vi "Window-Stop funct acq dialogue.vi"(7 "Colour":u32(colorbox)=16777225, 8 "error in (no error)":errorcluster, 9 "Caption-Left button (Cancel)":string, 10 "Caption-Right button (OK)":string, 11 "Message string":string) -> (0 "error out":errorcluster, 1 "User canceled the Abort Or the func acqcompleted":bool, 3 "Funct acq completed":bool)   [LabVIEW 2013]
uses:
  <vilib>/Utility/miscctls.llb/LVPointTypeDef.ctl
  Typedefs/Set Main VI cursor.ctl
  Global Variables/General Globals.vi
panel:
  in  "Left Button":bool
  in  "Rigth Button":bool
  out "Message":string
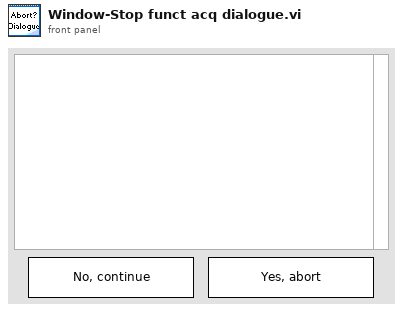
[diagram p1: front panel]
types:
  T1 = typedef "Set Main VI cursor.ctl" = enum16{"Release busy cursor", "Set busy cursor"}
  T2 = typedef "LVPointTypeDef.ctl" = cluster{"Horizontal":i16, "Vertical":i16}
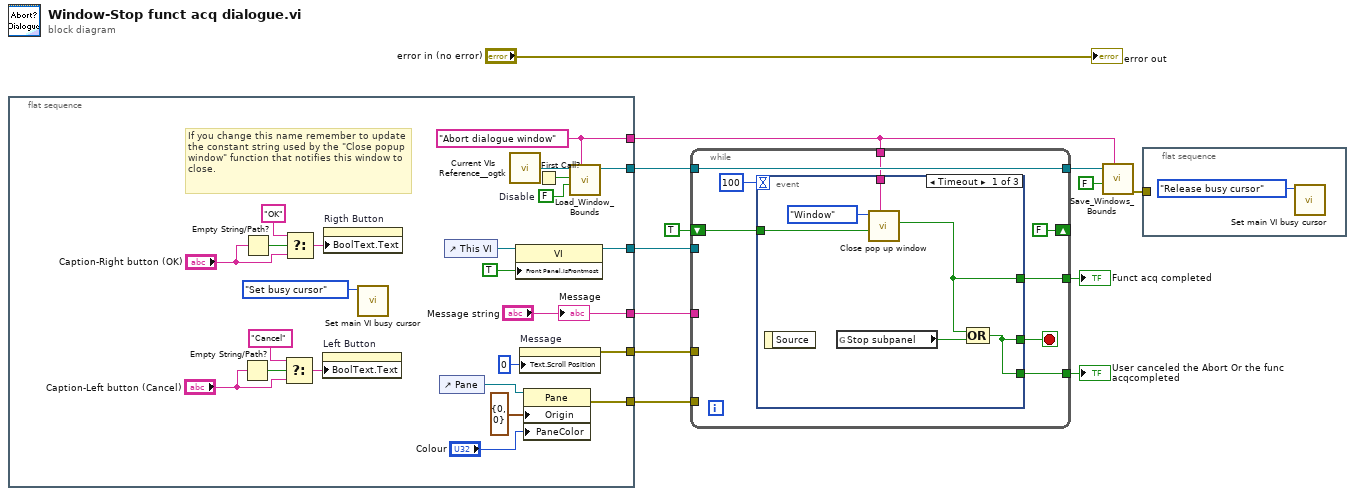
[diagram p0: block diagram]
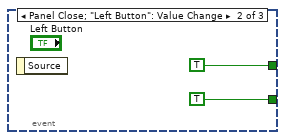
[diagram p2: hidden frame]
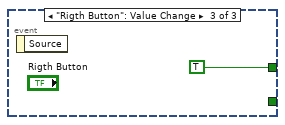
[diagram p3: hidden frame]
diagram:
  n1 = flat-sequence {
    tunnel: ["Message string"] -> w13
    tunnel: [w35] -> w12
    tunnel: [w32] -> w11
    tunnel: [w30] -> w10
    tunnel: [w25] -> w3
    tunnel: [w24] -> w7
    frame #0 {
      w26 = FALSE  # Disable
      w25 = "Abort dialogue window" ("Window Name (i.e. Key)")
      # "If you change this name remember to update the constant string used by the \"Close popup window\" function that notifies this window to close."
      n2 = Empty String/Path?(string/path="Caption-Left button (Cancel)") -> (empty?=w18:bool)
      n3 = Empty String/Path?(string/path="Caption-Right button (OK)") -> (empty?=w22:bool)
      n4 = Select(t="Cancel", s=w18, f="Caption-Left button (Cancel)") -> (s? t:f=w17:string)
      n5 = Select(t="OK", s=w22, f="Caption-Right button (OK)") -> (s? t:f=w20:string)
      n6 = property on="Left Button" class="Bool"("BoolText.Text"=w17) -> ()  [unwired: 2 in, 2 out]
      n7 = property on="Rigth Button" class="Bool"("BoolText.Text"=w20) -> ()  [unwired: 2 in, 2 out]
      n8 = call "Set main VI busy cursor.vi"("Main VI's cursor"=Set_Main_VI_cursor."Set busy cursor") -> ()  [unwired: 10 in, 1 out]
      n9 = control-ref of="Pane"() -> (w29:refnum<vi>)
      n10 = control-ref of="This VI"() -> (w33:refnum<vi>)
      n11 = call "Current VIs Reference__ogtk.vi"() -> ("Current VI's reference"=w28:refnum<vi>)  [unwired: 5 in]
      n12 = property on="Property Node" class="VI"(reference=w33, "Front Panel.IsFrontmost"=TRUE ("Front Panel Window:Is Frontmost")) -> (reference out=w32:refnum<vi>)  [unwired: 1 in, 1 out]
      n13 = property on="Message" class="Str"("Text.Scroll Position"=u32 0) -> (error out=w35:errorcluster)  [unwired: 2 in, 1 out]
      n14 = property class="Pane"(reference=w29, "Origin"=T2 {"Horizontal"=0, "Vertical"=0}, "PaneColor"="Colour") -> (error out=w30:errorcluster)  [unwired: 1 in, 1 out]
      n15 = First Call?() -> (First Call?: T/F=w27:bool)
      n16 = call "Load_Window_Bounds.vi"("Window Name (i.e. Key)"=w25, "Disable"=w26, "First Call"=w27, "Window VI's Ref"=w28) -> ("reference out"=w24:refnum<vi>)  [unwired: 4 in, 3 out]
      "Message" <- "Message string"
    }
  }
  n17 = while {
    tunnel: w13 -> [_]
    tunnel: w12 -> [_]
    tunnel: w10 -> [_]
    tunnel: w11 -> [_]
    tunnel: [w43] -> w9
    tunnel: w7 -> [w42]
    tunnel: [w42] -> w6
    shift-right: [FALSE] -> _
    shift-left: TRUE -> [w39]
    tunnel: w3 -> [w40]
    tunnel: [w38] -> w2
    stop <- w45 stop-if-true
    n18 = event shown="[0] Timeout" {
      selector: _ -> [_ _ _]
      dyn-events: _ -> [_ _ _]
      timeout: 100 -> [_ _ _]
      tunnel: [w46 TRUE ("Stop?") TRUE ("Stop?")] -> w45
      tunnel: [w46 TRUE ("Stop subpanel") _] -> w43
      tunnel: w40 -> [w50 _ _]
      tunnel: w39 -> [w49 _ _]
      tunnel: [w47 _ _] -> w38
      event Timeout {
        n19 = event-data() -> ()  [unwired: 1 in, 1 out]
        n20 = global read "General Globals.vi" "Stop subpanel"() -> (w48:bool)
        n21 = call "Close pop up window.vi"("Notifier's name"=w50, "Initialise"=w49, "Location"=enum16{"Window", "Process"}."Window") -> ("Stop window's loop (use this to close the window)"=w47:bool)  [unwired: 6 in, 2 out]
        n22 = Compound Arithmetic op=OR(w47, w48) -> (w46:bool)
      }
      event Panel Close; "Left Button": Value Change {
        n23 = event-data() -> ()  [unwired: 1 in, 1 out]
      }
      event "Rigth Button": Value Change {
        n24 = event-data() -> ()  [unwired: 1 in, 1 out]
      }
    }
  }
  "User canceled the Abort Or the func acqcompleted" <- w9
  "Funct acq completed" <- w2
  n25 = call "Save_Windows_Bounds.vi"("Window Name (i.e. Key)"=w3, "Front Panel Window:Open"=FALSE, "Window VI's Ref"=w6) -> ("Error out (pass-through)"=w1:errorcluster)  [unwired: 8 in]
  n26 = flat-sequence {
    tunnel: w1 -> [_]
    frame #0 {
      n27 = call "Set main VI busy cursor.vi"("Main VI's cursor"=Set_Main_VI_cursor."Release busy cursor") -> ()  [unwired: 10 in, 1 out]
    }
  }
  "error out" <- "error in (no error)"
